vi "Trigger Delay Driver Test.vi"() -> ()   [LabVIEW 2016]
uses:
  Ni-Scope Digitizer.lvclass
  C:/github/NHMFL_Core/Libraries/Instruments/Pulse Driver/Pulse Driver.lvclass
  Instruments/Pulse Driver/Pusle Driver Configuration.ctl
  Ni-Scope Digitizer.lvclass/Ni-Scope Digitizer.ctl
  Instruments/Pulse Driver/Pulse Driver.lvclass/Pulse Driver.ctl
  Write Device name.vi
  Instruments/Pulse Driver/Read t0.vi
  Instruments/Pulse Driver/Read dt.vi
  Instruments/Pulse Driver/Read Scaling coefficients.vi
  Instruments/Pulse Driver/Write Pulse Configuration.vi
panel:
  in  "Fetch:Fetch Relative To 2":i32(ring)=482 items=["Start"=482, "Trigger"=483, "Pretrigger"=477, "Now"=481, "Read Pointer"=388]
  in  "Read I16?":bool
  out "Fetch:Fetch Relative To":i32(ring)=482 items=["Start"=482, "Trigger"=483, "Pretrigger"=477, "Now"=481, "Read Pointer"=388]
  out "Fetch:Fetch Offset":i32
  out "Finished":bool
  in  "vertical range":dbl=10.0 format="%.2f"
  in  "min record length":i32=100000
  in  "reference position":dbl=50.0 format="%.1f"
  in  "min sample rate":dbl=1000000.0 format="%^.2e"
  in  "channels":string="0"
  in  "resource name":refnum<k15>="5105-PCI"
  out "Waveform Graph":waveform(dbl)[](graph)
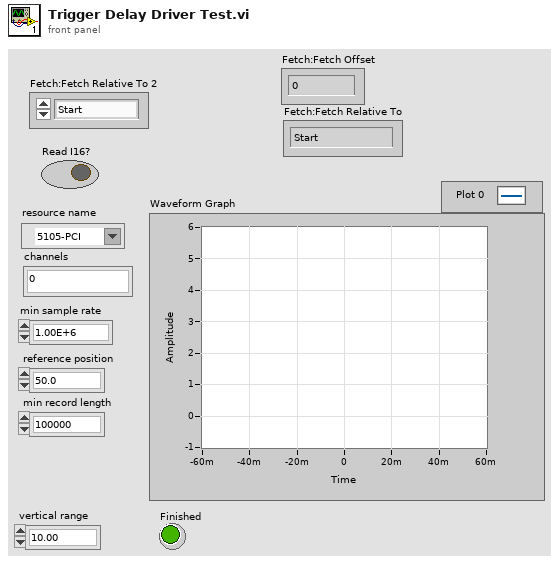
[diagram p1: front panel]
types:
  T1 = typedef "Pusle Driver Configuration.ctl" = cluster{"Pre-trigger duration":dbl, "Post-trigger duration":dbl, "Rate":dbl, "Ranges":dbl[], "Re-name channels":string[], "Active channels":string, "External clock":bool}
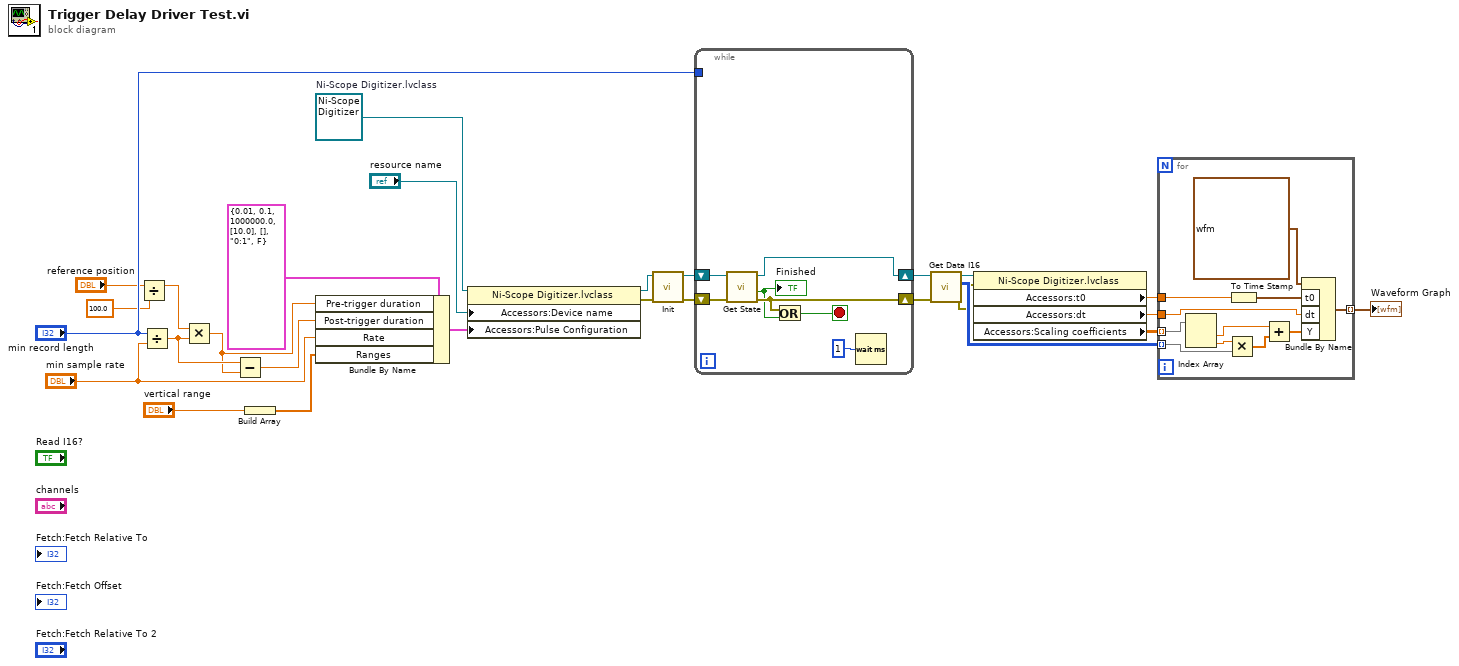
[diagram p0: block diagram]
diagram:
  w26 = refnum<class "Ni-Scope Digitizer.lvclass"> refnum  # Ni-Scope Digitizer.lvclass
  n1 = Divide(x="reference position", y=100.0) -> (x/y=w2:dbl)
  n2 = Divide(x="min record length", y="min sample rate") -> (x/y=w17:dbl)
  n3 = Multiply(x=w2, y=w17) -> (x*y=w16:dbl)
  n4 = Subtract(x=w17, y=w16) -> (x-y=w15:dbl)
  n5 = Build Array("vertical range") -> (w21:dbl[])
  n6 = Bundle By Name(cluster=T1 {"Pre-trigger duration"=0.01, "Post-trigger duration"=0.1, "Rate"=1000000.0, "Ranges"=[10.0], "Re-name channels"=[], "Active channels"="0:1", "External clock"=FALSE} ("Pulse Configuration"), "Pre-trigger duration"=w16, "Post-trigger duration"=w15, "Rate"="min sample rate", "Ranges"=w21) -> (w23:T1)
  n7 = property class="Ni-Scope Digitizer.lvclass"(reference=w26, "Accessors:Device name"="resource name", "Accessors:Pulse Configuration"=w23) -> (reference out=w14:refnum<class "Ni-Scope Digitizer.lvclass">, error out=w13:errorcluster)  [unwired: 1 in]
  n8 = call-dynamic "Init.vi"("error in (no error)"=w13, "Pulse Driver in"=w14) -> ("error out"=w3:errorcluster, "Pulse Driver out"=w12:refnum<class "Ni-Scope Digitizer.lvclass">)  [unwired: 7 in, 1 out]
  n9 = while {
    shift-right: [w30] -> w9
    shift-left: w3 -> [w31]
    shift-right: [w28] -> w11
    shift-left: w12 -> [w32]
    tunnel: "min record length" -> [_]
    stop <- w34 stop-if-true
    n10 = call-dynamic "Get State.vi"("error in (no error)"=w31, "NI-Scope Digitizer in"=w32) -> ("error out"=w30:errorcluster, "Data ready"=w29:bool, "NI-Scope Digitizer out"=w28:refnum<class "Ni-Scope Digitizer.lvclass">)  [unwired: 4 in, 3 out]
    "Finished" <- w29
    n11 = Or(x=w30, y=w29) -> (x .or. y?=w34:bool)
    n12 = Wait (ms)(milliseconds to wait=u32 1) -> ()  [unwired: 1 out]
  }
  n13 = call-dynamic "Get Data I16.vi"("error in (no error)"=w9, "Ni-Scope Digitizer in"=w11) -> ("error out"=w4:errorcluster, "Data out"=w10:i16[][], "Ni-Scope Digitizer out"=w8:refnum<class "Ni-Scope Digitizer.lvclass">)  [unwired: 5 in, 2 out]
  n14 = property class="Ni-Scope Digitizer.lvclass"(reference=w8, error in=w4) -> ("Accessors:t0"=w7:dbl, "Accessors:dt"=w6:dbl, "Accessors:Scaling coefficients"=w5:dbl[][])  [unwired: 2 out]
  n15 = for {
    tunnel: [w43] -> w27 mode=indexing
    tunnel: w10 -> [w42] mode=indexing
    tunnel: w7 -> [w39]
    tunnel: w6 -> [w38]
    tunnel: w5 -> [w37] mode=indexing
    n16 = Index Array(array=w37) -> (element #1=w36:dbl, element #2=w35:dbl)  [unwired: 2 in]
    n17 = Multiply(x=w35, y=w42) -> (x*y=w41:dbl[])
    n18 = To Time Stamp(1:w39) -> (0:w44:timestamp)
    n19 = Add(x=w36, y=w41) -> (x+y=w40:dbl[])
    n20 = Bundle By Name(cluster=waveform(dbl) {"t0"=timestamp(0 s since 1904-01-01), "dt"=0.0, "Y"=[]} ("wfm"), "t0"=w44, "dt"=w38, "Y"=w40) -> (w43:waveform(dbl))
  }
  "Waveform Graph" <- w27
